vi "PostScanAction.vi"(0 "Device en entrée":refnum<class "DAQ6363.lvclass"> caption="DNL_LabVIEW Object in", 5 "AcqComp":bool, 7 "ScanDev":bool caption="AcqComp", 11 "error in (no error)":errorcluster caption="entrée d'erreur (pas d'erreur)") -> (4 "Device en sortie":refnum<class "DAQ6363.lvclass"> caption="DNL_LabVIEW Object out", 6 "PostScanString":string, 15 "error out":errorcluster caption="sortie d'erreur")   [LabVIEW 2019, in "DAQ6363.lvclass"]
uses:
  DAQ6363.lvclass
  C:/Programmes Labview/LabscanV1A/DevicesClass/BaseDevice/BaseDevice.lvclass
  DAQ6363.lvclass/DAQ6363.ctl
  <userlib>/GenProg/ReadValByRefTask.vi
  <userlib>/GenProg/ReadValByRefBool.vi
  <resource>/objmgr/daqmx.rc
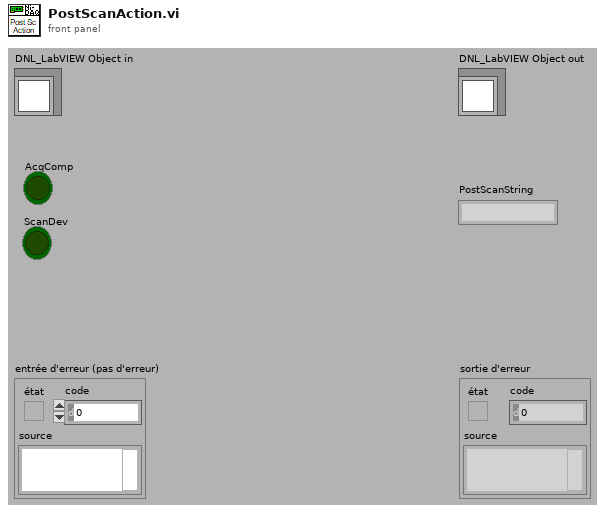
[diagram p1: front panel]
types:
  T1 = typedef "DAQ6363.lvclass/DAQ6363_Func.ctl" = enum16{"CountPulse (Cnt)", "Rabi (Tau)", "MWtoLaserDelay (us)", "APDGate (us)", "PulsedODMR (Pulses)"}
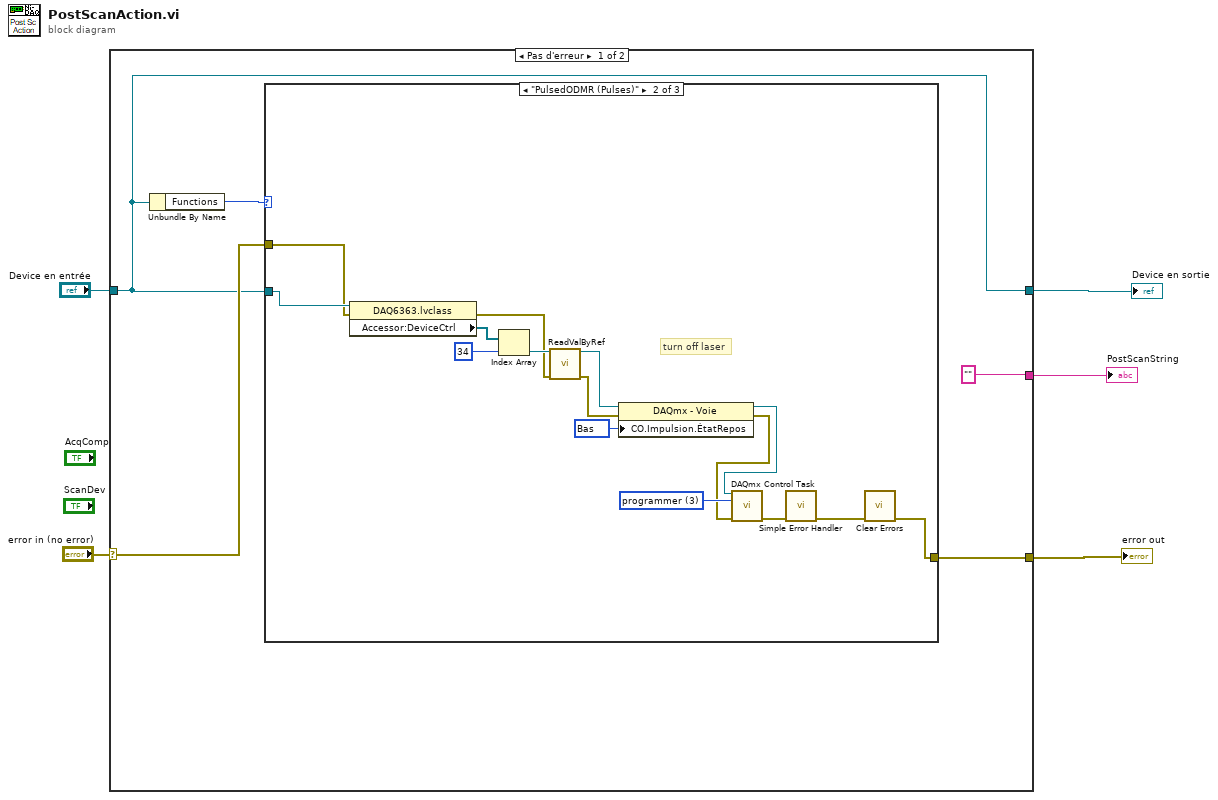
[diagram p0: block diagram]
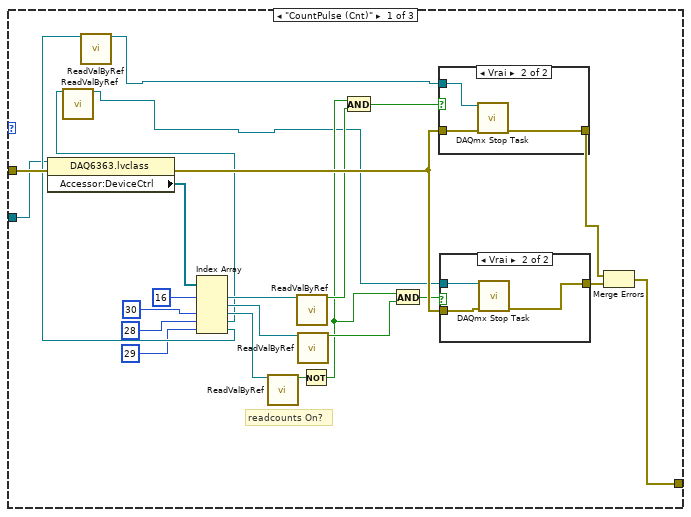
[diagram p2: hidden frame]
diagram:
  n1 = case shown="Pas d'erreur" "error in (no error)" {
    selector: "error in (no error)" -> [w9 w60]
    tunnel: [w8 w60] -> w1
    tunnel: [w6 w59] -> w4
    tunnel: "Device en entrée" -> [w6 w59]
    tunnel: ["" _] -> w3
    frame No Error {
      n2 = Unbundle By Name(w6) -> ("Functions"=w7:T1)
      n3 = case shown="\"PulsedODMR (Pulses)\"" w7 {
        tunnel: w9 -> [w26 w47 w58]
        tunnel: [w22 w43 w58] -> w8
        tunnel: w6 -> [w13 w51 _]
        frame "CountPulse (Cnt)" {
          # "readcounts On?"
          n4 = property class="DAQ6363.lvclass"(reference=w13, error in=w26) -> (error out=w33:errorcluster, "Accessor:DeviceCtrl"=w34:refnum<vi>[])  [unwired: 1 out]
          n5 = Index Array(array=w34, index #1=16 ("indice"), index #3=30 ("indice"), index #4=28 ("indice"), index #5=29 ("indice")) -> (element #1=w24:refnum<vi>, element #2=w23:refnum<vi>, element #3=w20:refnum<vi>, element #4=w15:refnum<vi>, element #5=w14:refnum<vi>)  [unwired: 1 in]
          n6 = call-poly <userlib>:"ReadValByRef.vi"("Control Ref"=w15) -> ("Valeur"=w16:refnum<k21>)  [unwired: 13 in, 1 out]
          n7 = call-poly <userlib>:"ReadValByRef.vi"("Control Ref"=w14) -> ("Valeur"=w17:refnum<k21>)  [unwired: 13 in, 1 out]
          n8 = call-poly <userlib>:"ReadValByRef.vi"("Control Ref"=w20) -> ("Valeur"=w19:bool)  [unwired: 13 in, 1 out]
          n9 = call-poly <userlib>:"ReadValByRef.vi"("Control Ref"=w24) -> ("Valeur"=w30:bool)  [unwired: 13 in, 1 out]
          n10 = call-poly <userlib>:"ReadValByRef.vi"("Control Ref"=w23) -> ("Valeur"=w28:bool)  [unwired: 13 in, 1 out]
          n11 = Not(x=w19) -> (.not. x?=w18:bool)
          n12 = And(x=w18, y=w30) -> (x .and. y?=w29:bool)
          n13 = And(x=w18, y=w28) -> (x .and. y?=w27:bool)
          n14 = case shown="Vrai" w29 {
            tunnel: w17 -> [_ w42]
            tunnel: w33 -> [w39 w41]
            tunnel: [w39 w40] -> w31
            frame False {
            }
            frame True {
              n15 = call <vilib>:"DAQmx Stop Task.vi"("task/channels in"=w42, "error in"=w41) -> ("error out"=w40:errorcluster)  [unwired: 12 in, 1 out]
            }
          }
          n16 = case shown="Vrai" w27 {
            tunnel: w16 -> [_ w38]
            tunnel: w33 -> [w35 w37]
            tunnel: [w35 w36] -> w32
            frame False {
            }
            frame True {
              n17 = call <vilib>:"DAQmx Stop Task.vi"("task/channels in"=w38, "error in"=w37) -> ("error out"=w36:errorcluster)  [unwired: 12 in, 1 out]
            }
          }
          n18 = Merge Errors(w31, w32) -> (w22:errorcluster)
        }
        frame "PulsedODMR (Pulses)" {
          w56 = 3 items=["vérifier"=2, "réserver"=4, "programmer"=3, "libérer"=5, "abandonner"=6] ("action")
          w57 = 10214 items=["Haut"=10192, "Bas"=10214] ("CO.Impulsion.ÉtatRepos")
          # "turn off laser"
          n19 = property class="DAQ6363.lvclass"(reference=w51, error in=w47) -> (error out=w48:errorcluster, "Accessor:DeviceCtrl"=w53:refnum<vi>[])  [unwired: 1 out]
          n20 = Index Array(array=w53, index=34 ("indice")) -> (element=w49:refnum<vi>)
          n21 = call-poly <userlib>:"ReadValByRef.vi"("Control Ref"=w49, "error in"=w48) -> ("Valeur"=w50:refnum<k21>, "error out"=w46:errorcluster)  [unwired: 12 in]
          n22 = property class="DAQmx - Voie"(reference=w50, error in=w46, "CO.Impulsion.ÉtatRepos"=w57) -> (reference out=w55:refnum<k21>, error out=w54:errorcluster)
          n23 = call <vilib>:"DAQmx Control Task.vi"("task/channels in"=w55, "action"=w56, "error in"=w54) -> ("error out"=w45:errorcluster)  [unwired: 11 in, 1 out]
          n24 = call <vilib>:"Simple Error Handler.vi"("error in (no error)"=w45) -> ("error out"=w44:errorcluster)  [unwired: 4 in, 4 out]
          n25 = call <vilib>:"Clear Errors.vi"("error in (no error)"=w44) -> ("error out"=w43:errorcluster)  [unwired: 5 in, 1 out]
        }
        frame "Rabi (Tau)", Default {
        }
      }
    }
    frame Error {
    }
  }
  "error out" <- w1
  "Device en sortie" <- w4
  "PostScanString" <- w3
